vi "Terminal Relation Msg Input.vi"() -> (2 "Terminal Relation (Msg Input)":T1)   [LabVIEW 2025, in "_Rescript.lvlib" / "Msg.lvlib" / "Msg.lvclass"]
uses:
  Msg.lvclass
  Msg.lvclass/Msg.ctl
  Terminal Relation.ctl
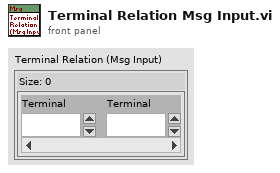
[diagram p1: front panel]
types:
  T1 = typedef "_Rescript.lvlib/Msg.lvlib/Msg.lvclass/Terminal Relation.ctl" = map{i32, i32}
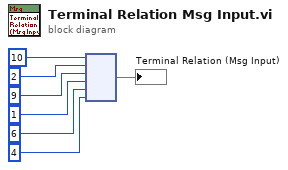
[diagram p0: block diagram]
diagram:
  n1 = node(10 ("Numeric"), 2 ("Numeric"), 9 ("Numeric"), 1 ("Numeric"), 6 ("key"), 4 ("value")) -> (→"Terminal Relation (Msg Input)":map{i32, i32})
